vi "single tp default data.vi"(1 "字符串":string) -> (0 "item data":string)   [LabVIEW 2018]
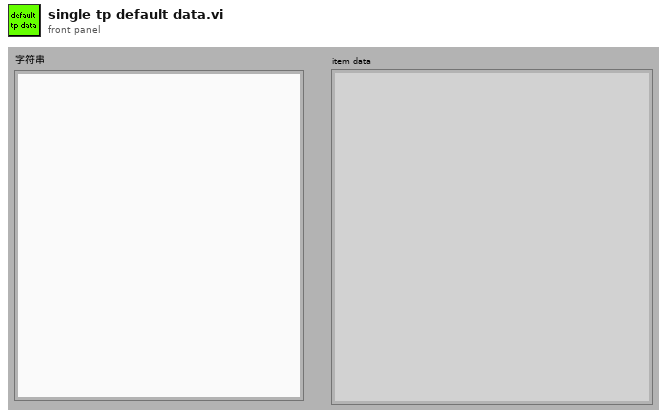
[diagram p1: front panel]
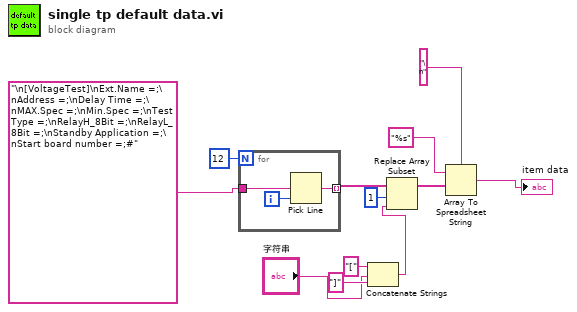
[diagram p0: block diagram]
diagram:
  n1 = for {
    N: 12 -> [_]
    tunnel: "\n[VoltageTest]\nExt.Name =;\nAddress =;\nDelay Time =;\nMAX.Spec =;\nMin.Spec =;\nTest Type =;\nRelayH_8Bit =;\nRelayL_8Bit =;\nStandby Application =;\nStart board number =;#" -> [w14]
    tunnel: [w15] -> w10 mode=indexing
    i -> [w13]
    n2 = Pick Line(multi-line string=w14, line index=w13) -> (output string=w15:string)  [unwired: 1 in]
  }
  n3 = Concatenate Strings("[" ("字符串"), "字符串", "]" ("字符串")) -> (w3:string)
  n4 = Replace Array Subset(array=w10, new element=w3, index=1 ("索引")) -> (w9:string[])
  n5 = Array To Spreadsheet String(delimiter (Tab)="\n" ("分隔符(Tab)"), array=w9, 3:"%s" ("格式字符串")) -> (spreadsheet string=→"item data":string)
